vi "SSH_Read.vi"(8 "error in (no error)":errorcluster, 11 "Python in":cluster{"Python":refnum<k35>, "py file":path}) -> (0 "error out":errorcluster, 2 "Reply":string, 3 "Python out":cluster{"Python":refnum<k35>, "py file":path})   [LabVIEW 2020]
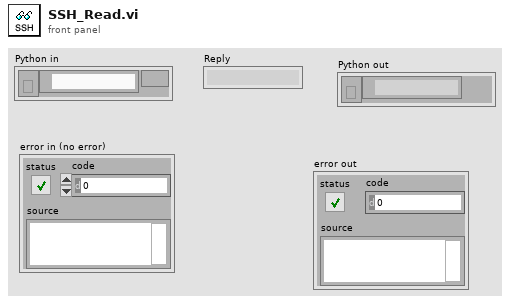
[diagram p1: front panel]
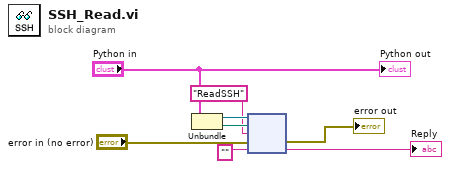
[diagram p0: block diagram]
diagram:
  n1 = Unbundle("Python in") -> ("Python"=w7:refnum<k35>, "py file"=w8:path)
  n2 = node(w7, w8, "ReadSSH" ("function name"), "error in (no error)", "" ("replace string (\"\")")) -> (→"error out":errorcluster, →"Reply":string)  [unwired: 3 out]
  "Python out" <- "Python in"
